vi "Hardware-CalPointConstants.vi"   [LabVIEW 2016, in "DSI-RT.lvlib"]
uses:
  DSI-RT.lvlib
  <vilib>/addons/Software Calibration Management/xSCM/CalPoint.xnode
  <vilib>/addons/Software Calibration Management/xSCM/ni_scm.dll
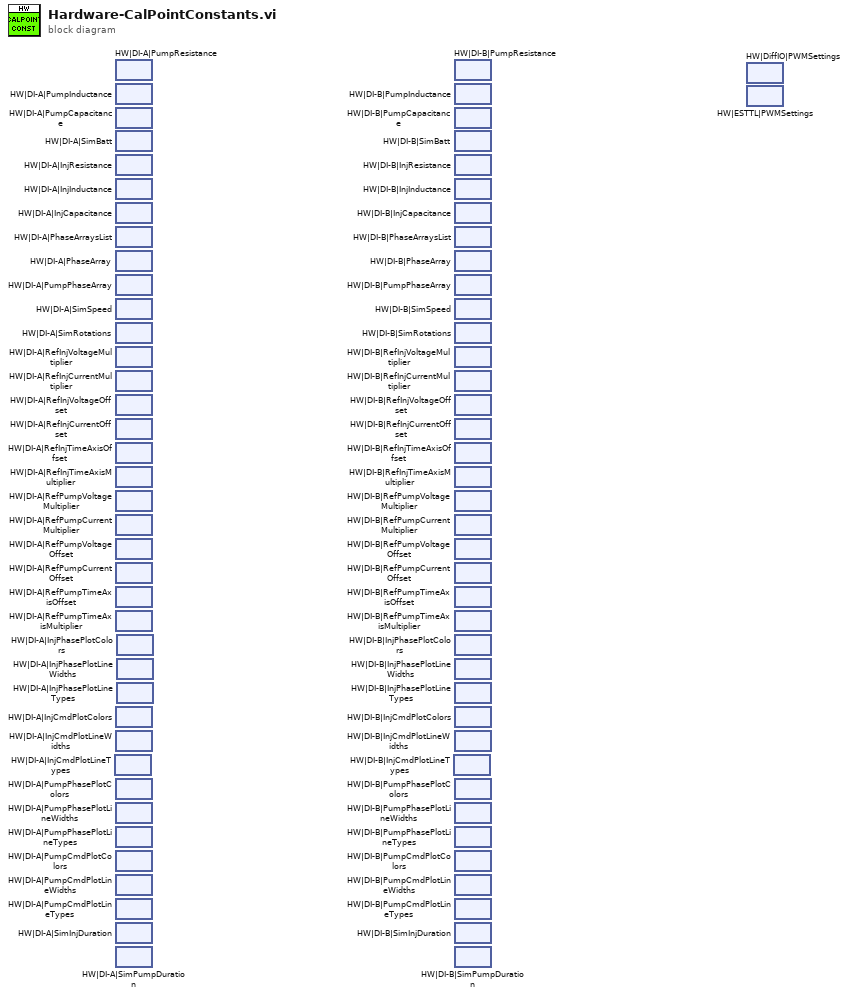
[diagram p0: block diagram]
diagram:
  n1 = xnode "HW|DI-A|InjCmdPlotLineTypes"() -> ()  [unwired: 1 out]
  n2 = xnode "HW|DI-A|PumpResistance"() -> ()  [unwired: 1 out]
  n3 = xnode "HW|DI-A|PumpInductance"() -> ()  [unwired: 1 out]
  n4 = xnode "HW|DI-A|PumpCapacitance"() -> ()  [unwired: 1 out]
  n5 = xnode "HW|DI-A|SimBatt"() -> ()  [unwired: 1 out]
  n6 = xnode "HW|DI-A|InjResistance"() -> ()  [unwired: 1 out]
  n7 = xnode "HW|DI-A|InjInductance"() -> ()  [unwired: 1 out]
  n8 = xnode "HW|DI-A|InjCapacitance"() -> ()  [unwired: 1 out]
  n9 = xnode "HW|DI-A|PhaseArraysList"() -> ()  [unwired: 1 out]
  n10 = xnode "HW|DI-A|PhaseArray"() -> ()  [unwired: 1 out]
  n11 = xnode "HW|DI-A|PumpPhaseArray"() -> ()  [unwired: 1 out]
  n12 = xnode "HW|DI-A|SimSpeed"() -> ()  [unwired: 1 out]
  n13 = xnode "HW|DI-A|SimRotations"() -> ()  [unwired: 1 out]
  n14 = xnode "HW|DI-A|RefInjVoltageMultiplier"() -> ()  [unwired: 1 out]
  n15 = xnode "HW|DI-A|RefInjCurrentMultiplier"() -> ()  [unwired: 1 out]
  n16 = xnode "HW|DI-A|RefInjVoltageOffset"() -> ()  [unwired: 1 out]
  n17 = xnode "HW|DI-A|RefInjCurrentOffset"() -> ()  [unwired: 1 out]
  n18 = xnode "HW|DI-A|RefInjTimeAxisOffset"() -> ()  [unwired: 1 out]
  n19 = xnode "HW|DI-A|RefInjTimeAxisMultiplier"() -> ()  [unwired: 1 out]
  n20 = xnode "HW|DI-A|RefPumpVoltageMultiplier"() -> ()  [unwired: 1 out]
  n21 = xnode "HW|DI-A|RefPumpCurrentMultiplier"() -> ()  [unwired: 1 out]
  n22 = xnode "HW|DI-A|RefPumpVoltageOffset"() -> ()  [unwired: 1 out]
  n23 = xnode "HW|DI-A|RefPumpCurrentOffset"() -> ()  [unwired: 1 out]
  n24 = xnode "HW|DI-A|RefPumpTimeAxisOffset"() -> ()  [unwired: 1 out]
  n25 = xnode "HW|DI-A|RefPumpTimeAxisMultiplier"() -> ()  [unwired: 1 out]
  n26 = xnode "HW|DI-A|InjCmdPlotColors"() -> ()  [unwired: 1 out]
  n27 = xnode "HW|DI-A|InjCmdPlotLineWidths"() -> ()  [unwired: 1 out]
  n28 = xnode "HW|DI-A|PumpPhasePlotColors"() -> ()  [unwired: 1 out]
  n29 = xnode "HW|DI-A|PumpPhasePlotLineWidths"() -> ()  [unwired: 1 out]
  n30 = xnode "HW|DI-A|PumpPhasePlotLineTypes"() -> ()  [unwired: 1 out]
  n31 = xnode "HW|DI-A|PumpCmdPlotColors"() -> ()  [unwired: 1 out]
  n32 = xnode "HW|DI-A|PumpCmdPlotLineWidths"() -> ()  [unwired: 1 out]
  n33 = xnode "HW|DI-A|PumpCmdPlotLineTypes"() -> ()  [unwired: 1 out]
  n34 = xnode "HW|DI-A|SimInjDuration"() -> ()  [unwired: 1 out]
  n35 = xnode "HW|DI-A|SimPumpDuration"() -> ()  [unwired: 1 out]
  n36 = xnode "HW|DI-A|InjPhasePlotColors"() -> ()  [unwired: 1 out]
  n37 = xnode "HW|DI-A|InjPhasePlotLineWidths"() -> ()  [unwired: 1 out]
  n38 = xnode "HW|DI-A|InjPhasePlotLineTypes"() -> ()  [unwired: 1 out]
  n39 = xnode "HW|DI-B|InjCmdPlotLineTypes"() -> ()  [unwired: 1 out]
  n40 = xnode "HW|DI-B|PumpResistance"() -> ()  [unwired: 1 out]
  n41 = xnode "HW|DI-B|PumpInductance"() -> ()  [unwired: 1 out]
  n42 = xnode "HW|DI-B|PumpCapacitance"() -> ()  [unwired: 1 out]
  n43 = xnode "HW|DI-B|SimBatt"() -> ()  [unwired: 1 out]
  n44 = xnode "HW|DI-B|InjResistance"() -> ()  [unwired: 1 out]
  n45 = xnode "HW|DI-B|InjInductance"() -> ()  [unwired: 1 out]
  n46 = xnode "HW|DI-B|InjCapacitance"() -> ()  [unwired: 1 out]
  n47 = xnode "HW|DI-B|PhaseArraysList"() -> ()  [unwired: 1 out]
  n48 = xnode "HW|DI-B|PhaseArray"() -> ()  [unwired: 1 out]
  n49 = xnode "HW|DI-B|PumpPhaseArray"() -> ()  [unwired: 1 out]
  n50 = xnode "HW|DI-B|SimSpeed"() -> ()  [unwired: 1 out]
  n51 = xnode "HW|DI-B|SimRotations"() -> ()  [unwired: 1 out]
  n52 = xnode "HW|DI-B|RefInjVoltageMultiplier"() -> ()  [unwired: 1 out]
  n53 = xnode "HW|DI-B|RefInjCurrentMultiplier"() -> ()  [unwired: 1 out]
  n54 = xnode "HW|DI-B|RefInjVoltageOffset"() -> ()  [unwired: 1 out]
  n55 = xnode "HW|DI-B|RefInjCurrentOffset"() -> ()  [unwired: 1 out]
  n56 = xnode "HW|DI-B|RefInjTimeAxisOffset"() -> ()  [unwired: 1 out]
  n57 = xnode "HW|DI-B|RefInjTimeAxisMultiplier"() -> ()  [unwired: 1 out]
  n58 = xnode "HW|DI-B|RefPumpVoltageMultiplier"() -> ()  [unwired: 1 out]
  n59 = xnode "HW|DI-B|RefPumpCurrentMultiplier"() -> ()  [unwired: 1 out]
  n60 = xnode "HW|DI-B|RefPumpVoltageOffset"() -> ()  [unwired: 1 out]
  n61 = xnode "HW|DI-B|RefPumpCurrentOffset"() -> ()  [unwired: 1 out]
  n62 = xnode "HW|DI-B|RefPumpTimeAxisOffset"() -> ()  [unwired: 1 out]
  n63 = xnode "HW|DI-B|RefPumpTimeAxisMultiplier"() -> ()  [unwired: 1 out]
  n64 = xnode "HW|DI-B|InjPhasePlotColors"() -> ()  [unwired: 1 out]
  n65 = xnode "HW|DI-B|InjPhasePlotLineWidths"() -> ()  [unwired: 1 out]
  n66 = xnode "HW|DI-B|InjPhasePlotLineTypes"() -> ()  [unwired: 1 out]
  n67 = xnode "HW|DI-B|InjCmdPlotColors"() -> ()  [unwired: 1 out]
  n68 = xnode "HW|DI-B|InjCmdPlotLineWidths"() -> ()  [unwired: 1 out]
  n69 = xnode "HW|DI-B|PumpPhasePlotColors"() -> ()  [unwired: 1 out]
  n70 = xnode "HW|DI-B|PumpPhasePlotLineWidths"() -> ()  [unwired: 1 out]
  n71 = xnode "HW|DI-B|PumpPhasePlotLineTypes"() -> ()  [unwired: 1 out]
  n72 = xnode "HW|DI-B|PumpCmdPlotColors"() -> ()  [unwired: 1 out]
  n73 = xnode "HW|DI-B|PumpCmdPlotLineWidths"() -> ()  [unwired: 1 out]
  n74 = xnode "HW|DI-B|PumpCmdPlotLineTypes"() -> ()  [unwired: 1 out]
  n75 = xnode "HW|DI-B|SimInjDuration"() -> ()  [unwired: 1 out]
  n76 = xnode "HW|DI-B|SimPumpDuration"() -> ()  [unwired: 1 out]
  n77 = xnode "HW|DiffIO|PWMSettings"() -> ()  [unwired: 1 out]
  n78 = xnode "HW|ESTTL|PWMSettings"() -> ()  [unwired: 1 out]
